vi "Auto Index_recipe.vi"(11 "New Recipe.Para":T2(array[cluster])) -> (3 "Array":T1(array[cluster]))   [LabVIEW 2014, in "Master.lvclass"]
uses:
  Master/Master.lvclass
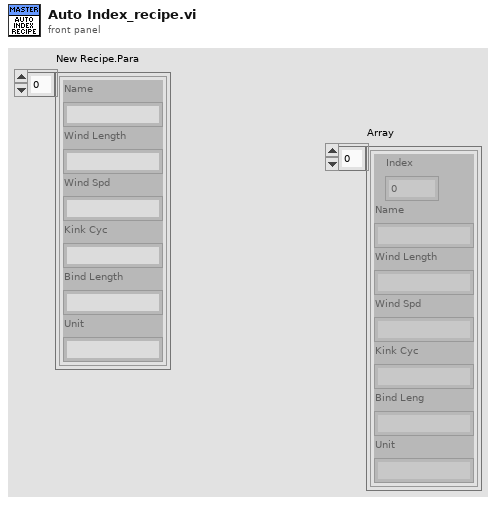
[diagram p1: front panel]
types:
  T1 = cluster{"Index":i32, "Name":string, "Wind Length":string, "Wind Spd":string, "Kink Cyc":string, "Bind Leng":string, "Unit":string}[]
  T2 = cluster{"Name":string, "Wind Length":string, "Wind Spd":string, "Kink Cyc":string, "Bind Length":string, "Unit":string}[]
  T3 = cluster{"Index":i32, "Name":string, "Wind Length":string, "Wind Spd":string, "Kink Cyc":string, "Bind Leng":string, "Unit":string}
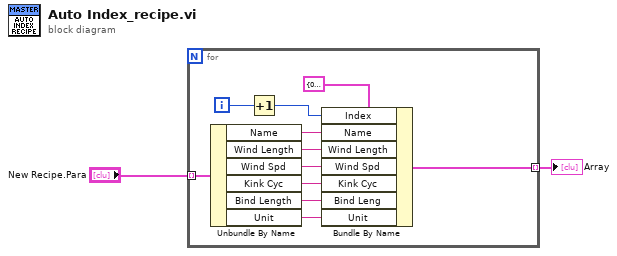
[diagram p0: block diagram]
diagram:
  n1 = for {
    tunnel: "New Recipe.Para" -> [w13] mode=indexing
    tunnel: [w3] -> w1 mode=indexing
    i -> [w12]
    n2 = Unbundle By Name(w13) -> ("Name"=w9:string, "Wind Length"=w8:string, "Wind Spd"=w7:string, "Kink Cyc"=w6:string, "Bind Length"=w5:string, "Unit"=w4:string)
    n3 = Increment(x=w12) -> (x+1=w10:i32)
    n4 = Bundle By Name(cluster=T3 {"Index"=0, "Name"="", "Wind Length"="", "Wind Spd"="", "Kink Cyc"="", "Bind Leng"="", "Unit"=""}, "Index"=w10, "Name"=w9, "Wind Length"=w8, "Wind Spd"=w7, "Kink Cyc"=w6, "Bind Leng"=w5, "Unit"=w4) -> (w3:T3)
  }
  "Array" <- w1
